vi "Write.vi"(8 "error in (no error)":errorcluster, 10 "Data":u8[](array[numeric])=[0], 11 "PCA in":refnum<class "PCA.lvclass">) -> (0 "error out":errorcluster, 3 "PCA out":refnum<class "PCA.lvclass">)   [LabVIEW 2022 SP3, in "PCA9685.lvlib" / "PCA.lvclass"]
uses:
  PCA.lvclass
  PCA.lvclass/PCA.ctl
  <vilib>/MakerHub/LINX/LMH-LINX.lvlib
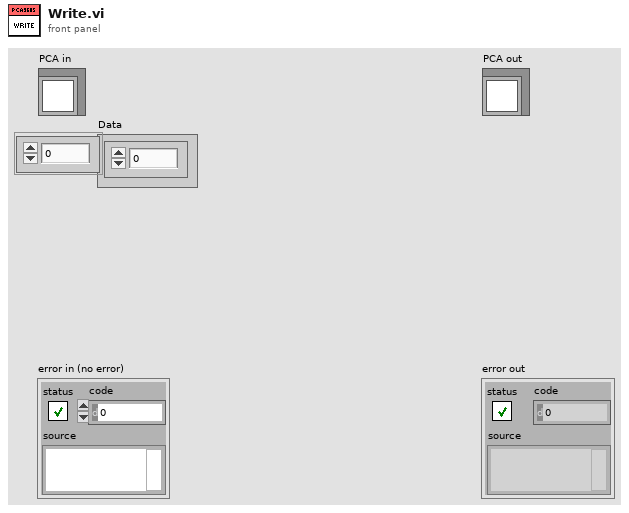
[diagram p1: front panel]
types:
  T1 = typedef "LMH-LINX.lvlib/LINX Ref.ctl" = cluster{"IO":T2, "Interface":T3, "LINX Device Config":T4}
  T2 = typedef "LMH-LINX.lvlib/Platform.ctl" = enum16{"Remote", "Local"}
  T3 = typedef "LMH-LINX.lvlib/Interface.ctl" = enum16{"Serial", "TCP"}
  T4 = typedef "LMH-LINX.lvlib/Device.lvlib/LINX Device Config.ctl" = cluster{"Interface":T3, "COM Port":refnum<visa-resource-name>, "TCP Configuration":T5, "Device Family":u8, "Device ID":u8, "Device Name":string, "TCP Ref":refnum<k5>, "Channels":T6}
  T5 = typedef "LMH-LINX.lvlib/Device.lvlib/TCP Config.ctl" = cluster{"IP Address":string, "Port":u16}
  T6 = typedef "LMH-LINX.lvlib/Channels.ctl" = cluster{"DI":u8[], "DO":u8[], "AI":u8[], "AO":u8[], "PWM":u8[], "QE":u8[], "UART":u8[], "I2C 2":u8[], "SPI":u8[], "CAN":u8[], "Servo":u8[], "AI Ref (V)":dbl, "AI Resolution (Bits)":u8, "AO Ref (V)":dbl, "AO Resolution (Bits)":u8}
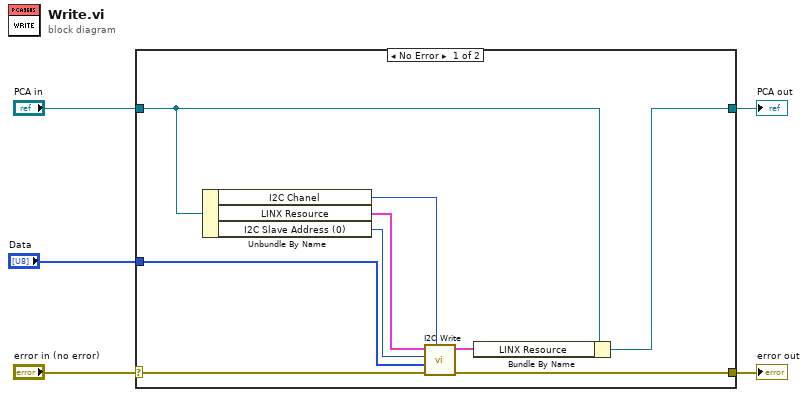
[diagram p0: block diagram]
diagram:
  n1 = case shown="No Error" "error in (no error)" {
    selector: "error in (no error)" -> [w10 w16]
    tunnel: [w11 w16] -> w4
    tunnel: [w13 w15] -> w2
    tunnel: "PCA in" -> [w14 w15]
    tunnel: "Data" -> [w9 _]
    frame No Error {
      n2 = Unbundle By Name(w14) -> ("I2C Chanel"=w6:u16, "LINX Resource"=w7:T1, "I2C Slave Address (0)"=w8:u16)
      n3 = call <vilib>:"I2C Write.vi"("I2C Channel"=w6, "Error In"=w10, "Data"=w9, "I2C Slave Address (0)"=w8, "LINX Resource"=w7) -> ("Error Out"=w11:errorcluster, "LINX Resource"=w12:T1)  [unwired: 5 in]
      n4 = Bundle By Name(cluster=w14, "LINX Resource"=w12) -> (w13:refnum<class "PCA.lvclass">)
    }
    frame Error {
    }
  }
  "error out" <- w4
  "PCA out" <- w2
